vi "VCS Get Gateway Settings.vi"(8 "error in (no error)":errorcluster, 11 "keyHandle in":u32) -> (0 "error out":errorcluster, 2 "baudrate":u32, 3 "keyHandle out":u32)   [LabVIEW 2010]
doc: "<B>VCS Get Gateway Settings</B> returns the baud rate and timeout gateway communication parameters"
uses:
  Resources/EposCmd64.dll
  Resources/EposCmd.dll
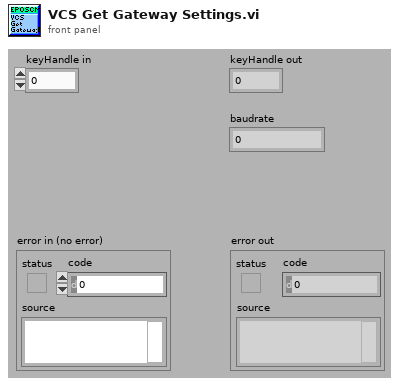
[diagram p1: front panel]
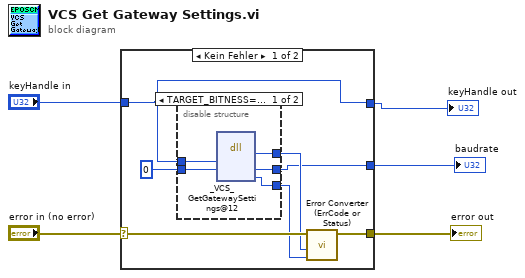
[diagram p0: block diagram]
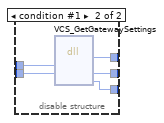
[diagram p2: hidden frame]
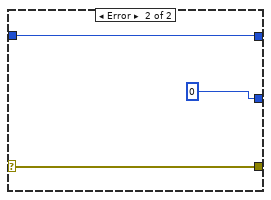
[diagram p3: hidden frame]
diagram:
  n1 = case shown="Kein Fehler" "error in (no error)" {
    selector: "error in (no error)" -> [w12 w25]
    tunnel: [w11 w25] -> w4
    tunnel: "keyHandle in" -> [w8 w24]
    tunnel: [w8 w24] -> w2
    tunnel: [w6 u32 0 ("pTimeout")] -> w1
    frame No Error {
      n2 = disable-structure shown="TARGET_BITNESS==32, Standard" {
        disable-tunnel: [w17 w22] -> w10
        disable-tunnel: u32 0 ("pBaudrate") -> [w16 w21]
        disable-tunnel: [w15 w20] -> w6
        disable-tunnel: w8 -> [w14 w19]
        disable-tunnel: [w13 w18] -> w7
        frame condition #0 (active) {
          n3 = dll-call lib="C:/Sources/LabVIEW/maxon EPOS/Resources/EposCmd.*" fn="_VCS_GetGatewaySettings@12" ("EposCmd.dll:_VCS_GetProtocolStackSettings@16")("KeyHandle"=w14, "pBaudrate"=w16) -> ("Rückgabetyp"=w13:i32, "pBaudrate"=w15:u32, "pErrorCode"=w17:u32)  [unwired: 5 in, 2 out]
        }
        frame condition #1 {
          n4 = dll-call lib="C:/Sources/LabView/maxon EPOS/Resources/EposCmd64.dll" fn="VCS_GetGatewaySettings" ("EposCmd.dll:_VCS_GetProtocolStackSettings@16")("KeyHandle"=w19, "pBaudrate"=w21) -> ("return type"=w18:i32, "pBaudrate"=w20:u32, "pErrorCode"=w22:u32)  [unwired: 5 in, 2 out]
        }
      }
      n5 = call "Error Converter (ErrCode or Status).vi"("error code"=w10, "return type"=w7, "error in (no error)"=w12) -> ("error out"=w11:errorcluster)  [unwired: 7 in]
    }
    frame Error {
    }
  }
  "error out" <- w4
  "keyHandle out" <- w2
  "baudrate" <- w1
